vi "Mouse Move.vi"(7 "Map Model in":refnum<class "Map Model.lvclass">, 8 "error in (no error)":errorcluster, 10 "Position":T1, 11 "Set Origin in":refnum<class "Set Origin.lvclass">) -> (0 "error out":errorcluster, 3 "Set Origin out":refnum<class "Set Origin.lvclass">, 5 "Map Model out":refnum<class "Map Model.lvclass">)   [LabVIEW 2020, in "Map Model.lvlib" / "Set Origin.lvclass"]
uses:
  Set Origin.lvclass
  <vilib>/Utility/miscctls.llb/LVPoint32TypeDef.ctl
  Map Model/Map Model.lvclass
  Map Model/Map Model.lvclass/Map Model.ctl
  Undoable Tool/Undoable Tool.lvclass
panel:
  # "NOTICE -- YOU MUST LEAVE THIS NOTICE IN PLACE.\n\nCopyright (c) 2017, LIANG LIU Shawn.Liu.cn@gmail.com\nAll rights reserved.\n\nRedistribution and use in source and binary forms, with or without modification, are permitted provided that the following conditions are met:\n-Redistributions of source code must retain the above copyright notice, this list of conditions and the following disclaimer.\n-Redistributions in binary form must reproduce the above copyright notice, this list of conditions and the following disclaimer in the documentation and/or other materials provided with the distribution.\n-Neither the name of the eLp nor the names of its contributors may be used to endorse or promote products derived from this software without specific prior written permission.\n\nTHIS SOFTWARE IS PROVIDED BY THE COPYRIGHT HOLDERS AND CONTRIBUTORS \"AS IS\" AND ANY EXPRESS OR IMPLIED WARRANTIES, INCLUDING, BUT NOT LIMITED TO, THE IMPLIED WARRANTIES OF MERCHANTABILITY AND FITNESS FOR A PARTICULAR PURPOSE ARE DISCLAIMED. IN NO EVENT SHALL THE COPYRIGHT HOLDER OR CONTRIBUTORS BE LIABLE FOR ANY DIRECT, INDIRECT, INCIDENTAL, SPECIAL, EXEMPLARY, OR CONSEQUENTIAL DAMAGES (INCLUDING, BUT NOT LIMITED TO, PROCUREMENT OF SUBSTITUTE GOODS OR SERVICES; LOSS OF USE, DATA, OR PROFITS; OR BUSINESS INTERRUPTION) HOWEVER CAUSED AND ON ANY THEORY OF LIABILITY, WHETHER IN CONTRACT, STRICT LIABILITY, OR TORT (INCLUDING NEGLIGENCE OR OTHERWISE) ARISING IN ANY WAY OUT OF THE USE OF THIS SOFTWARE, EVEN IF ADVISED OF THE POSSIBILITY OF SUCH DAMAGE."
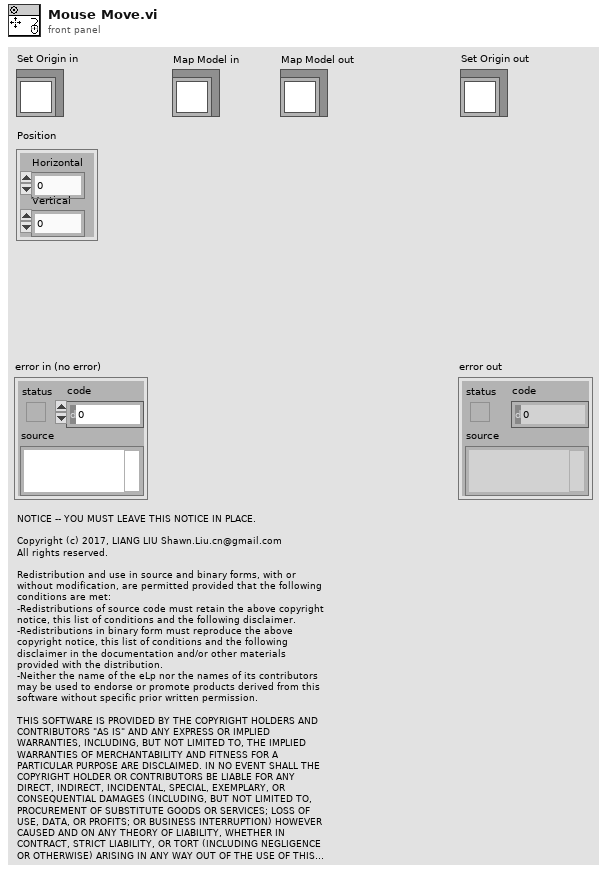
[diagram p1: front panel]
types:
  T1 = typedef "LVPoint32TypeDef.ctl" = cluster{"Horizontal":i32, "Vertical":i32}
  T2 = typedef "LVPointTypeDef.ctl" = cluster{"Horizontal":i16, "Vertical":i16}
  T3 = cluster{"Occupied Color":cluster{"Value":u8, "Color":u32}, "Free Color":cluster{"Value":u8, "Color":u32}, "Unknown Color":cluster{"Value":u8, "Color":u32}}
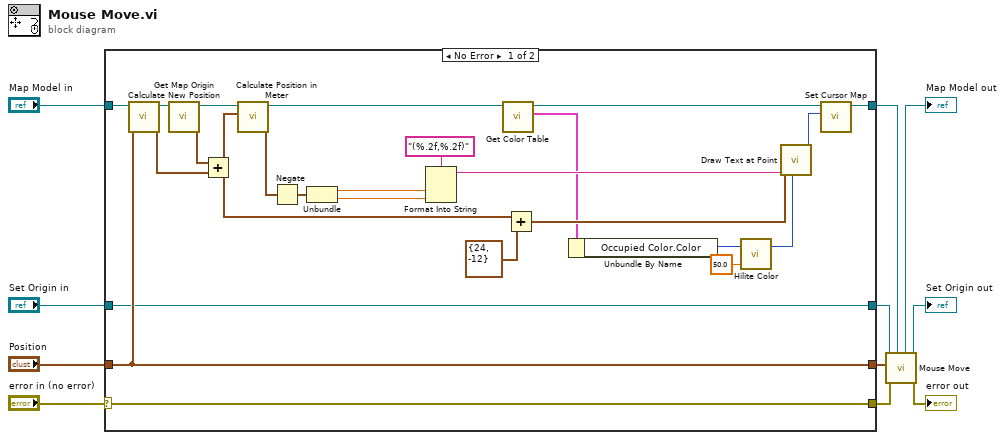
[diagram p0: block diagram]
diagram:
  n1 = case shown="No Error" "error in (no error)" {
    selector: "error in (no error)" -> [w35 w40]
    tunnel: "Map Model in" -> [w36 w37]
    tunnel: "Position" -> [w14 w39]
    tunnel: [w12 w37] -> w11
    tunnel: [w35 w40] -> w10
    tunnel: [w14 w39] -> w9
    tunnel: "Set Origin in" -> [w13 w38]
    tunnel: [w13 w38] -> w8
    frame No Error {
      n2 = call "Calculate New Position.vi"("Position in"=w14, "Map Model in"=w36) -> ("Position out"=w32:T1, "Map Model out"=w33:refnum<class "Map Model.lvclass">)  [unwired: 8 in]
      n3 = call "Get Map Origin.vi"("Map Model in"=w33) -> ("Map Origin"=w34:T2, "Map Model out"=w21:refnum<class "Map Model.lvclass">)  [unwired: 9 in]
      n4 = Add(x=w34, y=w32) -> (x+y=w18:T1)
      n5 = call "Calculate Position in Meter.vi"("Position on Map"=w18, "Map Model in"=w21) -> ("Position on PGM (m)"=w17:cluster{"Horizontal":dbl, "Vertical":dbl}, "Map Model out"=w20:refnum<class "Map Model.lvclass">)  [unwired: 8 in]
      n6 = Negate(x=w17) -> (-x=w26:cluster{"Horizontal":dbl, "Vertical":dbl})
      n7 = Unbundle(w26) -> ("Horizontal"=w29:dbl, "Vertical"=w28:dbl)
      n8 = Format Into String(format string="(%.2f,%.2f)", w29, w28) -> (resulting string=w27:string)  [unwired: 2 in, 1 out]
      n9 = call "Get Color Table.vi"("Map Model in"=w20) -> ("Color Table"=w23:T3, "Map Model out"=w19:refnum<class "Map Model.lvclass">)  [unwired: 9 in]
      n10 = Add(x=w18, y=T1 {"Horizontal"=24, "Vertical"=-12}) -> (x+y=w31:T1)
      n11 = Unbundle By Name(w23) -> ("Occupied Color.Color"=w22:u32)
      n12 = call <vilib>:"Hilite Color.vi"("Percentage(30)"=50.0, "Color In"=w22) -> ("Hilite"=w24:u32)  [unwired: 1 out]
      n13 = call <vilib>:"Draw Text at Point.vi"("text color(black)"=w24, "text"=w27, "origin"=w31) -> ("new picture"=w15:picture)  [unwired: 7 in, 1 out]
      n14 = call "Set Cursor Map.vi"("Cursor Map"=w15, "Map Model in"=w19) -> ("Map Model out"=w12:refnum<class "Map Model.lvclass">)  [unwired: 9 in]
    }
    frame Error {
    }
  }
  n15 = call-parent "Mouse Move.vi"("Map Model in"=w11, "error in (no error)"=w10, "Position"=w9, "Tool in"=w8) -> ("error out"=→"error out":errorcluster, "Tool out"=→"Set Origin out":refnum<class "Set Origin.lvclass">, "Map Model out"=→"Map Model out":refnum<class "Map Model.lvclass">)  [unwired: 5 in]
